vi "Check and Create File.vi"(8 "error in":errorcluster, 11 "Data Cluster In":T1={"UI Reference"={"All Ctrl's Label's"=[], "ChannelListTree"=refnum, "All Object Ref"=[]}, "Tree Selection"={"Selected Channel"="", "Selected Interface"="", "Selected HW"="", "Tree Root Name"=""}, "Selected File Path"=path "", "Selected HW"={"Slctd Hw Name"=[], "Slctd HW IP"=[]}, "Channel Config Path"=path "", "Interface Data"={"DO Channel's"=[]}, "General Info's"={"Idnentification name"=""}, "Status"="", "Channel Type's"={"Channel Type"=enum."Voltage", "Sub-Type"=enum."Pressure"}, "This VI"=refnum, "Hardware Information "=variant(variant[] [])}) -> (0 "error out":errorcluster, 2 "Read File?":bool, 3 "Data Cluster Out":T1={"UI Reference"={"All Ctrl's Label's"=[], "ChannelListTree"=refnum, "All Object Ref"=[]}, "Tree Selection"={"Selected Channel"="", "Selected Interface"="", "Selected HW"="", "Tree Root Name"=""}, "Selected File Path"=path "", "Selected HW"={"Slctd Hw Name"=[], "Slctd HW IP"=[]}, "Channel Config Path"=path "", "Interface Data"={"DO Channel's"=[]}, "General Info's"={"Idnentification name"=""}, "Status"="", "Channel Type's"={"Channel Type"=enum."Voltage", "Sub-Type"=enum."Pressure"}, "This VI"=refnum, "Hardware Information "=variant(variant[] [])})   [LabVIEW 2021, in "Configuration.lvlib"]
doc: "<b>Note:</b> This VI was modified by the <b>Validate DQMH Module</b> tool to turn off automatic error handling."
uses:
  Configuration.lvlib
  Module Data--cluster.ctl
  Host-Control's/Configuration UI Reference.ctl
  DO Channel's.ctl
  Config-Channel Type.ctl
  Channel Sub-Type.ctl
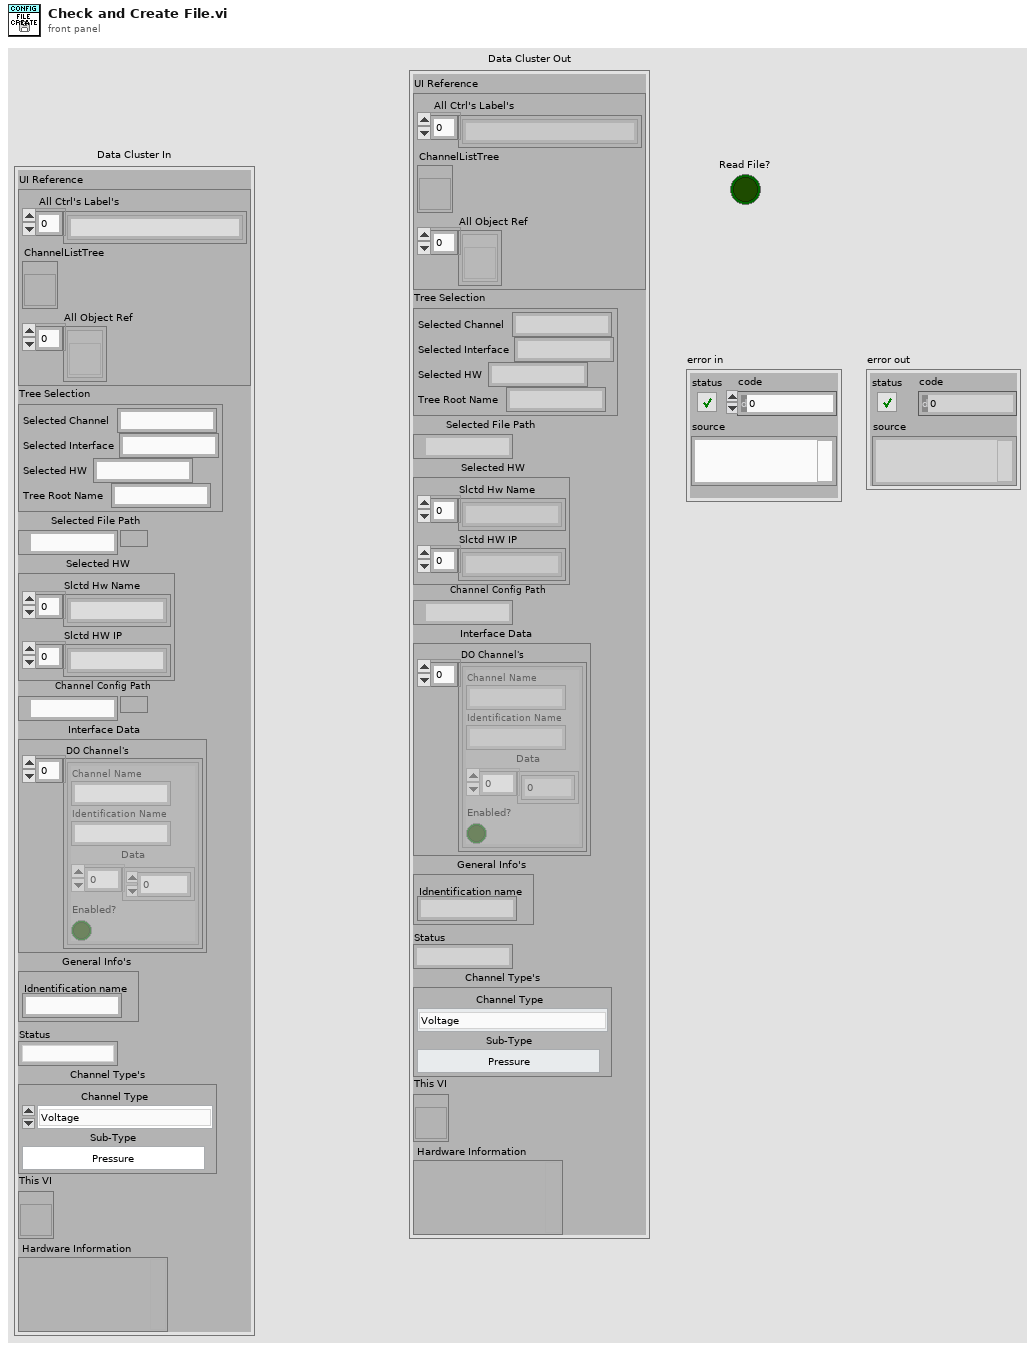
[diagram p1: front panel]
types:
  T1 = typedef "Configuration.lvlib/Module Data--cluster.ctl" = cluster{"UI Reference":T2, "Tree Selection":cluster{"Selected Channel":string, "Selected Interface":string, "Selected HW":string, "Tree Root Name":string}, "Selected File Path":path, "Selected HW":cluster{"Slctd Hw Name":string[], "Slctd HW IP":string[]}, "Channel Config Path":path, "Interface Data":cluster{"DO Channel's":T3}, "General Info's":cluster{"Idnentification name":string}, "Status":string, "Channel Type's":cluster{"Channel Type":T4, "Sub-Type":T5}, "This VI":refnum<vi>, "Hardware Information ":variant}
  T2 = typedef "Configuration UI Reference.ctl" = cluster{"All Ctrl's Label's":string[], "ChannelListTree":refnum<vi>, "All Object Ref":refnum<vi>[]}
  T3 = typedef "Configuration.lvlib/DO Channel's.ctl" = cluster{"Channel Name":string, "Identification Name":string, "Data":u8[], "Enabled?":bool}[]
  T4 = typedef "Configuration.lvlib/Config-Channel Type.ctl" = enum16{"Voltage", "Current", "Thermocouple", "Acclerometer"}
  T5 = typedef "Configuration.lvlib/Channel Sub-Type.ctl" = enum16{"None", "Pressure", "Force"}
  T6 = enum16{"open", "replace", "create", "open or create", "replace or create", "replace or create with confirmation"}
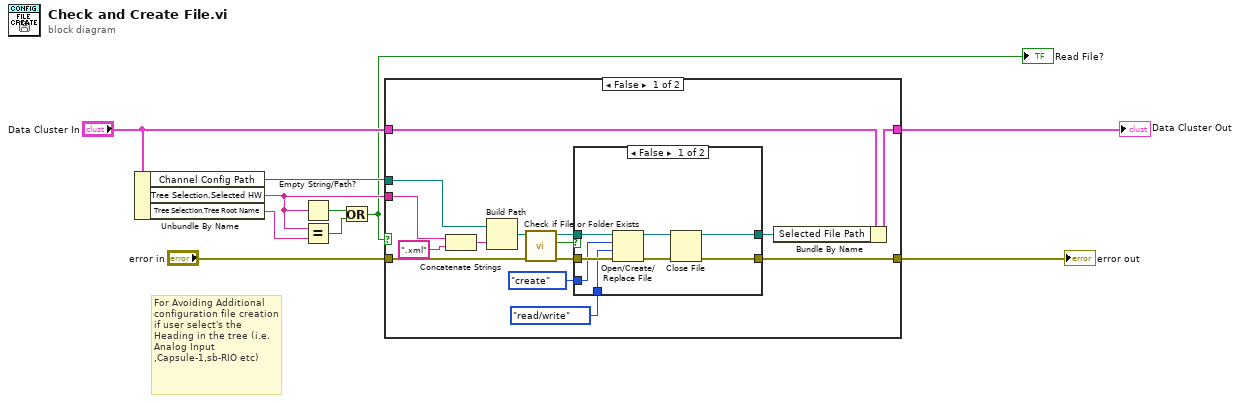
[diagram p0: block diagram]
diagram:
  # "For Avoiding Additional configuration file creation if user select's the Heading in the tree (i.e. Analog Input ,Capsule-1,sb-RIO etc)"
  n1 = Unbundle By Name("Data Cluster In") -> ("Channel Config Path"=w10:path, "Tree Selection.Selected HW"=w4:string, "Tree Selection.Tree Root Name"=w5:string)
  n2 = Empty String/Path?(string/path=w4) -> (empty?=w3:bool)
  n3 = Equal?(x=w4, y=w5) -> (x = y?=w2:bool)
  n4 = Or(x=w3, y=w2) -> (x .or. y?=w1:bool)
  "Read File?" <- w1
  n5 = case shown="False" w1 {
    tunnel: w10 -> [w25 _]
    tunnel: w4 -> [w14 _]
    tunnel: [w18 w37] -> w9
    tunnel: "error in" -> [w13 w37]
    tunnel: "Data Cluster In" -> [w17 w36]
    tunnel: [w16 w36] -> w6
    frame False {
      n6 = Concatenate Strings(w14, ".xml") -> (w19:string)
      n7 = Build Path(base path=w25, name or relative path=w19) -> (appended path=w24:path)
      n8 = call <vilib>:"Check if File or Folder Exists.vi"("error in (no error)"=w13, "path"=w24) -> ("error out"=w21:errorcluster, "file or folder exists?"=w23:bool, "dup path"=w22:path)  [unwired: 7 in]
      n9 = case shown="False" w23 {
        tunnel: w22 -> [w33 w35]
        tunnel: w21 -> [w32 w34]
        tunnel: [w28 w34] -> w18
        tunnel: [w29 w35] -> w15
        tunnel: enum16{"read/write", "read-only", "write-only"}."read/write" ("access (0:read/write)") -> [w27 _]
        tunnel: T6."create" ("operation (0:open)") -> [w26 _]
        frame False {
          n10 = Open/Create/Replace File(file path (use dialog)=w33, error in=w32, operation (0:open)=w26, access (0:read/write)=w27) -> (refnum out=w31:refnum<file>, error out=w30:errorcluster)  [unwired: 2 in, 1 out]
          n11 = Close File(refnum=w31, error in=w30) -> (path=w29:path, error out=w28:errorcluster)
        }
        frame True {
        }
      }
      n12 = Bundle By Name(cluster=w17, "Selected File Path"=w15) -> (w16:T1)
    }
    frame True {
    }
  }
  "Data Cluster Out" <- w6
  "error out" <- w9
